vi "hardware_close_hardware.vi"(8 "error in (no error)":errorcluster, 11 "galvo in":refnum<class "galvo.lvclass">) -> (0 "error out":errorcluster, 3 "galvo out":refnum<class "galvo.lvclass">)   [LabVIEW 2015, in "galvo.lvclass"]
uses:
  galvo.lvclass
  galvo.lvclass/galvo.ctl
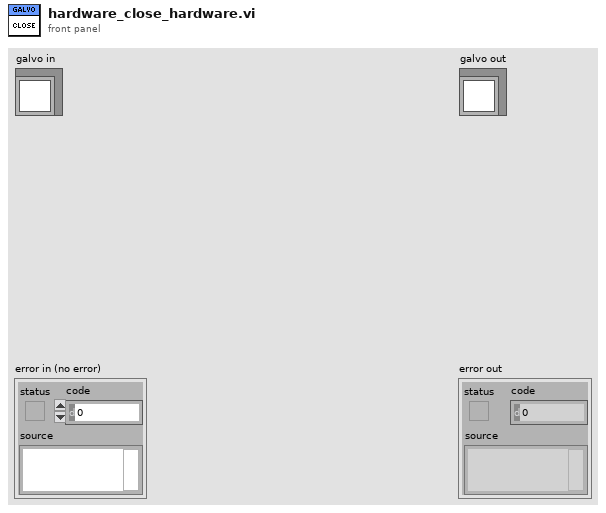
[diagram p1: front panel]
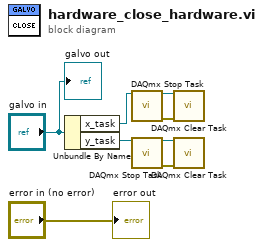
[diagram p0: block diagram]
diagram:
  n1 = Unbundle By Name("galvo in") -> ("x_task"=w8:refnum<k21>, "y_task"=w7:refnum<k21>)
  n2 = call <vilib>:"DAQmx Stop Task.vi"("task/channels in"=w8) -> ("task out"=w4:refnum<k21>, "error out"=w3:errorcluster)  [unwired: 13 in]
  n3 = call <vilib>:"DAQmx Stop Task.vi"("task/channels in"=w7) -> ("task out"=w6:refnum<k21>, "error out"=w5:errorcluster)  [unwired: 13 in]
  n4 = call <vilib>:"DAQmx Clear Task.vi"("task in"=w4, "error in"=w3) -> ()  [unwired: 13 in, 1 out]
  n5 = call <vilib>:"DAQmx Clear Task.vi"("task in"=w6, "error in"=w5) -> ()  [unwired: 13 in, 1 out]
  "error out" <- "error in (no error)"
  "galvo out" <- "galvo in"
